vi "Package Builder.vi"() -> ()   [LabVIEW 2019, in "VIPM.lvclass"]
uses:
  VIPM.lvclass
  <vilib>/Utility/sysdir.llb/System Directory Type.ctl
  <vilib>/Utility/file.llb/Read Delimited Spreadsheet (string).vi
  <vilib>/Utility/file.llb/Write Delimited Spreadsheet (string).vi
  <vilib>/JKI/VIPM API/VIPM API_vipm_api.lvlib
panel:
  out "Package Builder":string
  in  "Clear Notes":bool
  in  "Release Notes":string
  in  "Append Notes":bool
  in  "ALL":bool
  in  "Patch +1":bool
  out "Selected File List":string
  in  "Publish":bool
  in  "Open List":bool
  in  "Build":bool
  in  "Preview":bool
  out "Status":string
  in  "File List":i32(listbox)
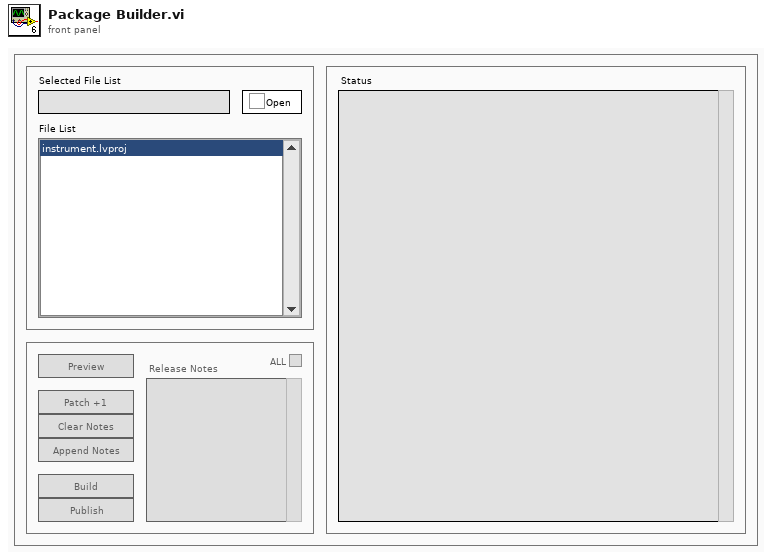
[diagram p1: front panel]
types:
  T1 = enum32{"Invalid", "Standard", "Closed", "Hidden", "Minimized", "Maximized"}
  T2 = enum32{"invalid app kind", "Development System", "Run Time System", "Student Edition", "Embedded LabVIEW", "Evaluation", "Custom"}
  T3 = enum8{"Enabled", "Disabled", "Disabled and Grayed Out"}
  T4 = cluster{"Core":cluster{"Current VI Reference":refnum<vi>, "Close Panel on Exit?":bool}, "lvproj paths":path[], "vipb paths":path[], "vip paths":path[], "selected path":path, "config path":path}
  T5 = typedef "System Directory Type.ctl" = i32
  T6 = cluster{"Current VI Reference":refnum<vi>, "Close Panel on Exit?":bool}
  T7 = typedef "VIPM API_vipm_api.lvlib/VI Package Build Spec Data Cluster_vipm_api.ctl" = cluster{"Package Version":T8, "Product Name":string, "Company Name":string, "Author Name (Person or Company)":string, "Product Homepage (URL)":string, "Legal Copyright":string, "License Agreement Name":string, "Product Description Summary":string, "Product Description":string, "Release Notes - Change Log":string}
  T8 = typedef "VIPM API_vipm_api.lvlib/Version Info Cluster_vipm_api.ctl" = cluster{"major":u32, "minor":u32, "patch":u32, "build":u32}
  T9 = typedef "VIPM API_vipm_api.lvlib/Repository Info Cluster_vipm_api.ctl" = cluster{"Repository Name":string, "Repository Folder Location":path}
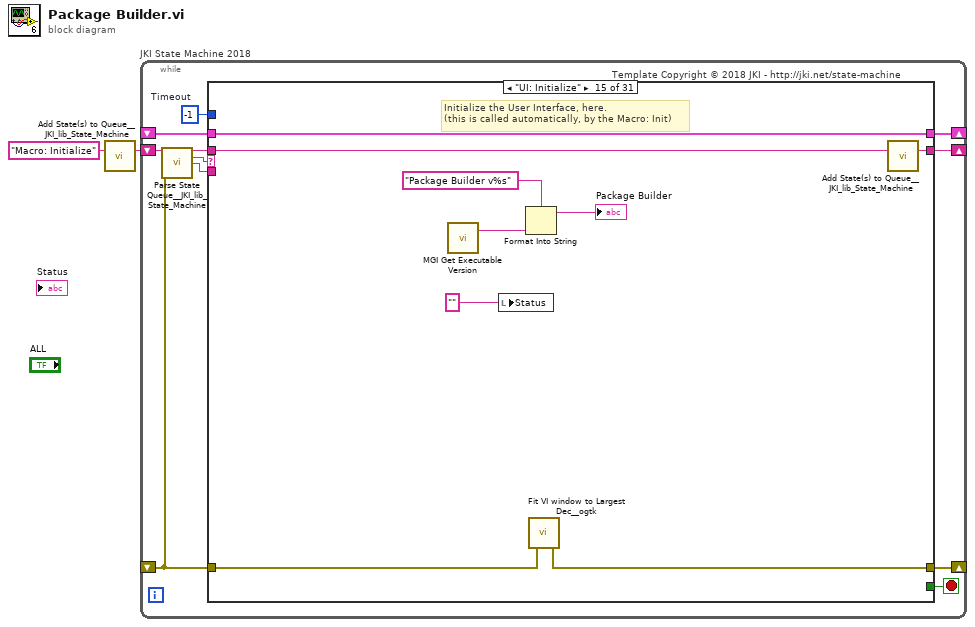
[diagram p0: block diagram]
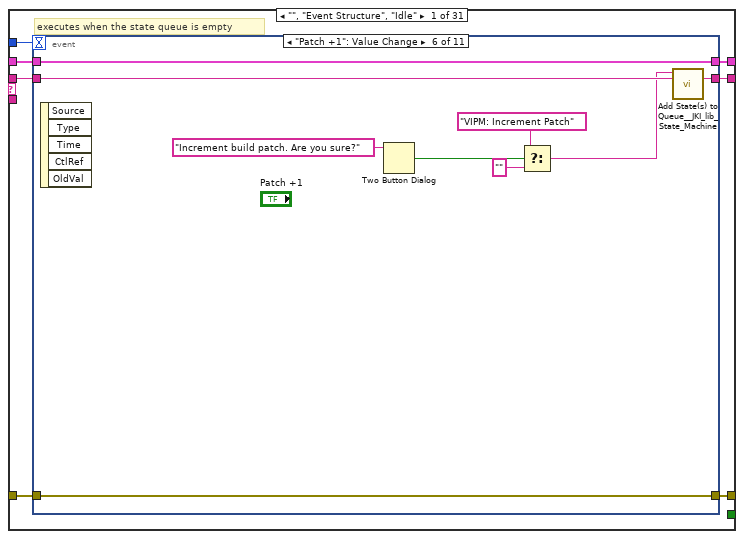
[diagram p2: hidden frame]
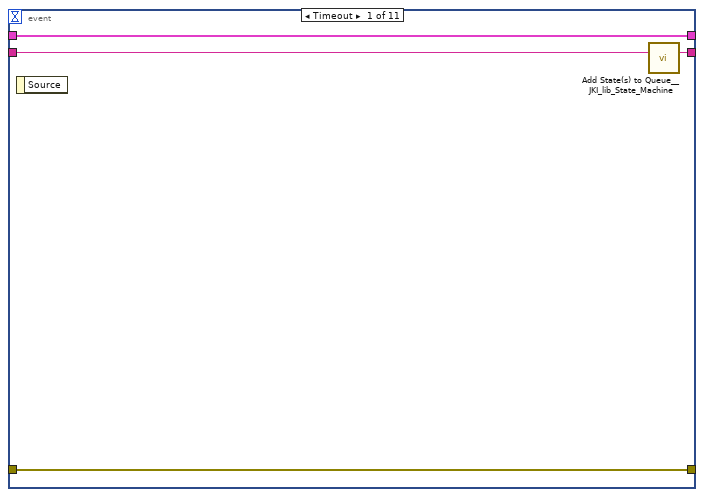
[diagram p3: hidden frame]
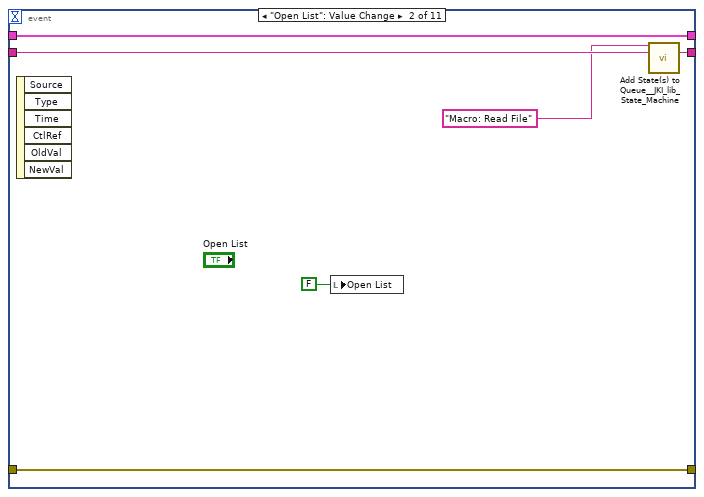
[diagram p4: hidden frame]
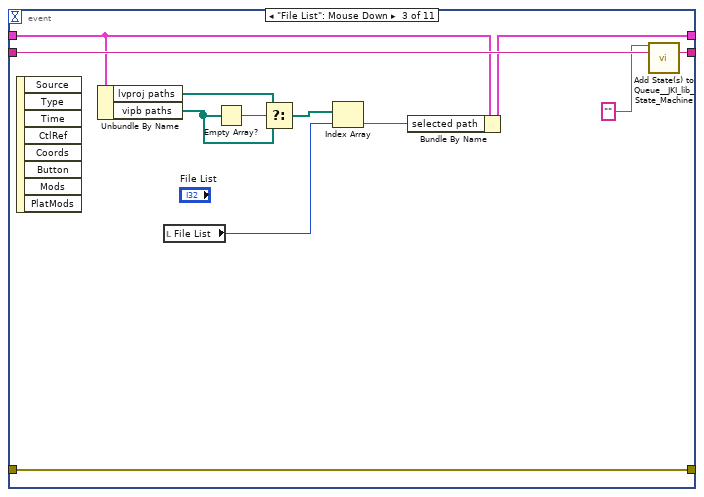
[diagram p5: hidden frame]
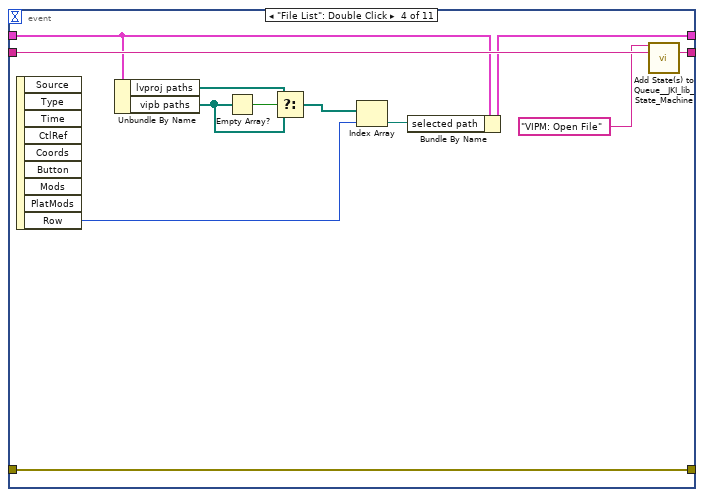
[diagram p6: hidden frame]
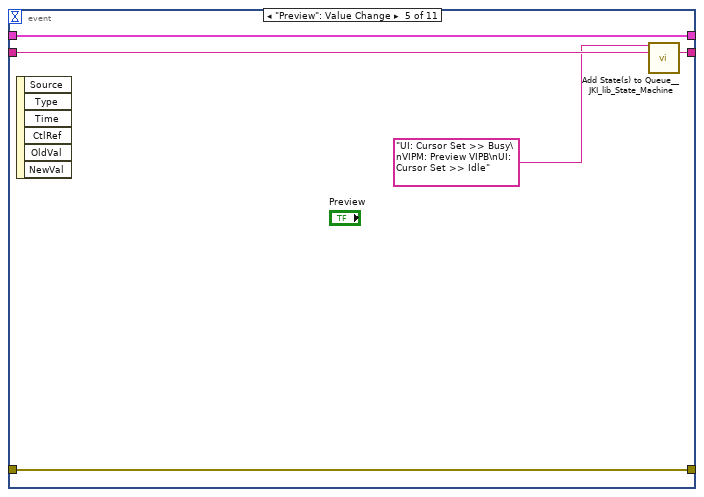
[diagram p7: hidden frame]
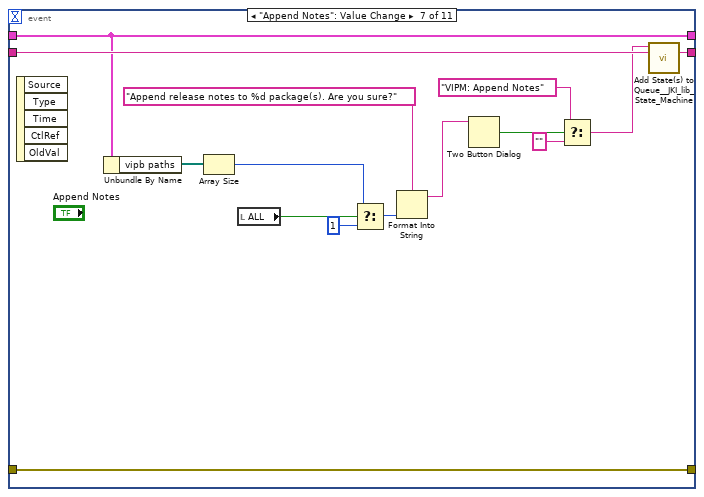
[diagram p8: hidden frame]
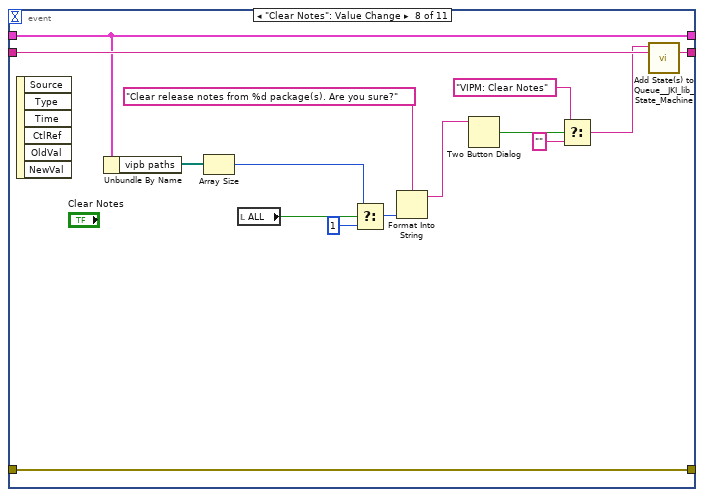
[diagram p9: hidden frame]
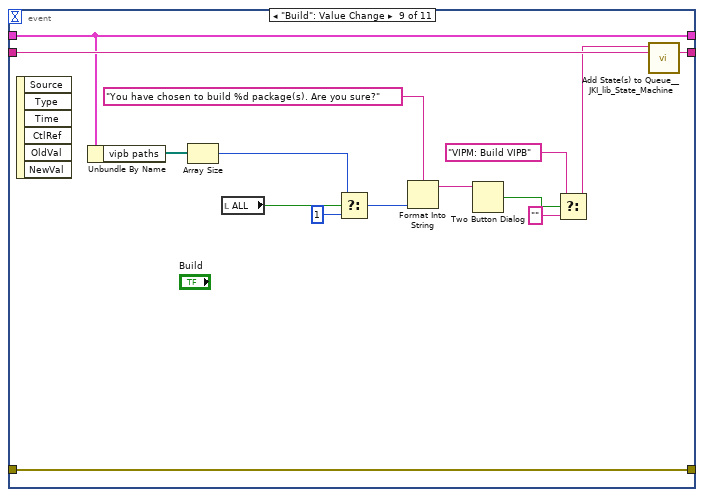
[diagram p10: hidden frame]
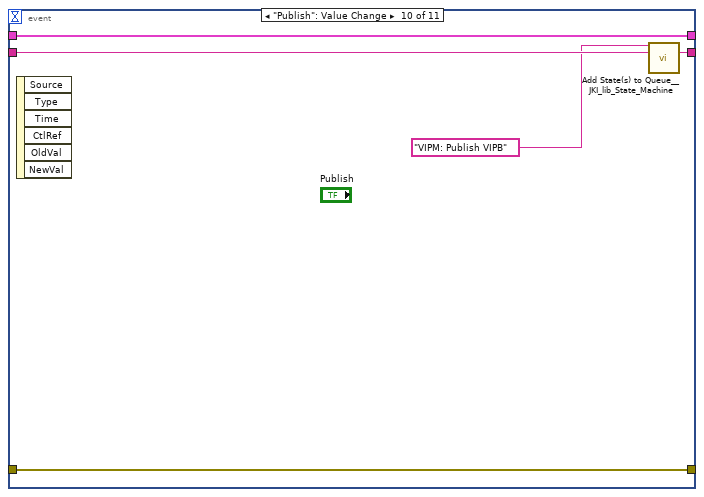
[diagram p11: hidden frame]
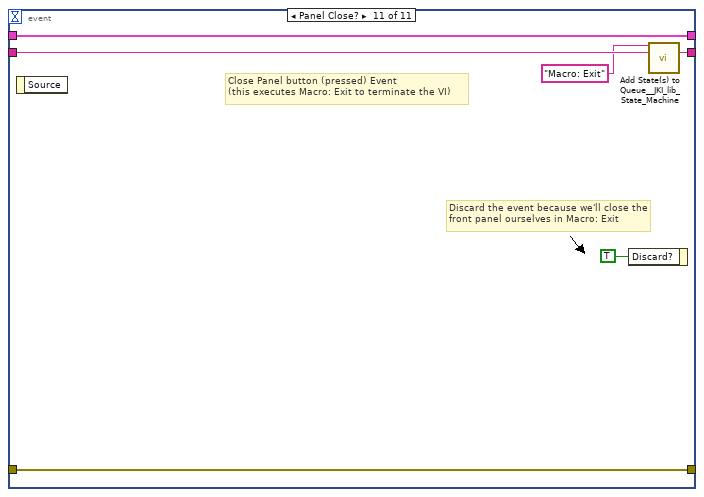
[diagram p12: hidden frame]
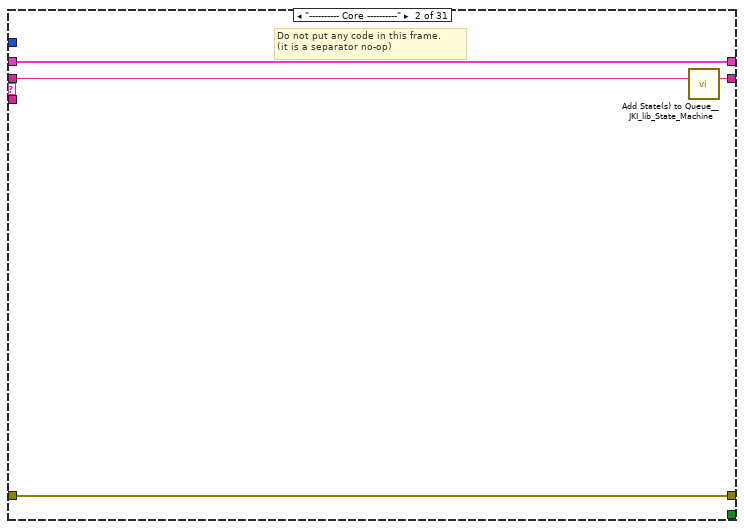
[diagram p13: hidden frame]
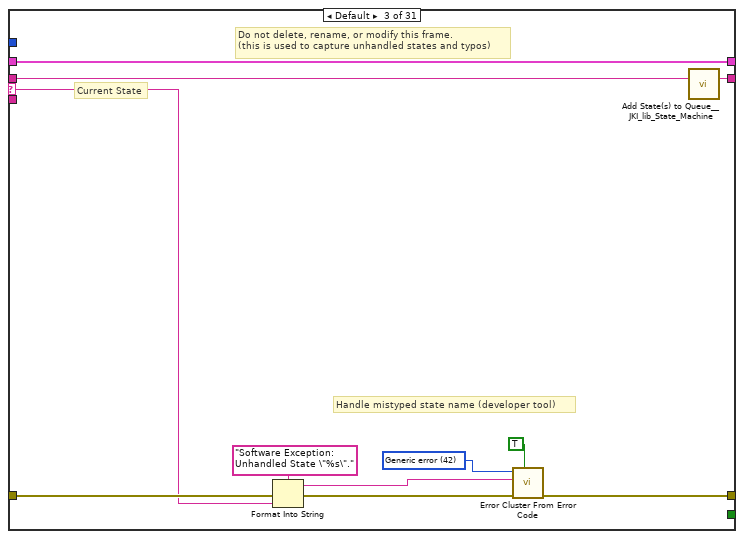
[diagram p14: hidden frame]
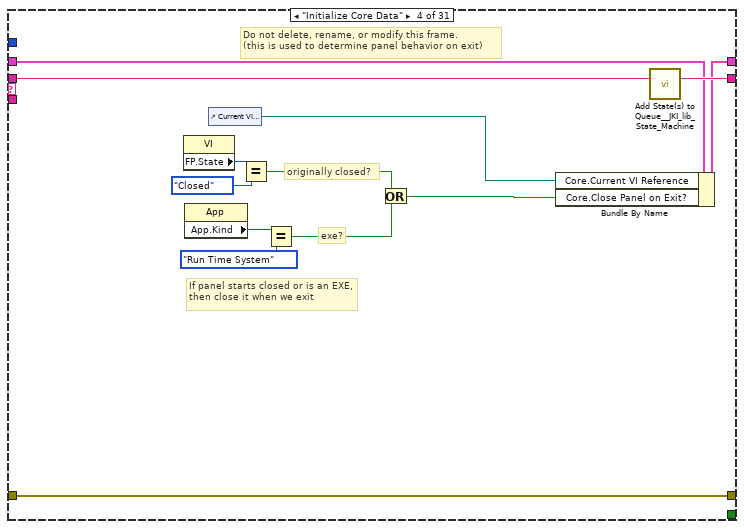
[diagram p15: hidden frame]
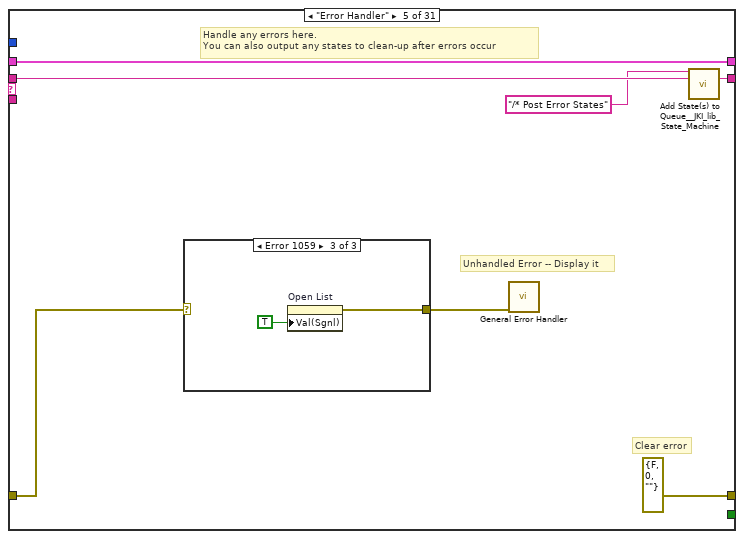
[diagram p16: hidden frame]
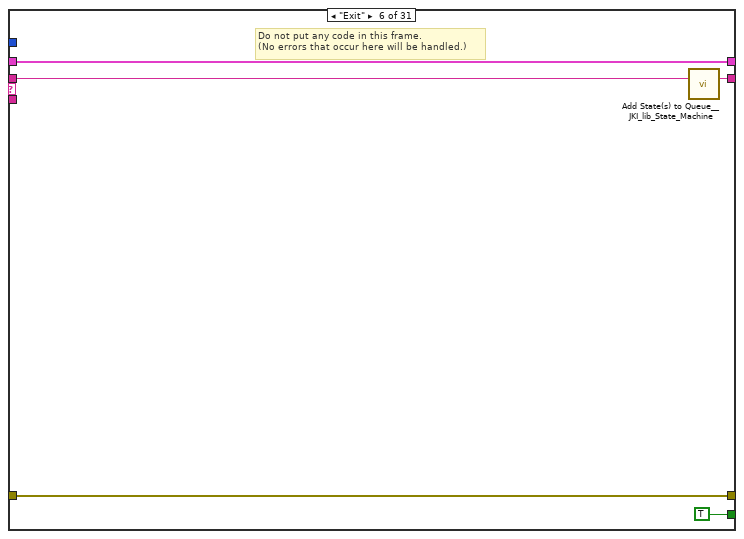
[diagram p19: hidden frame]
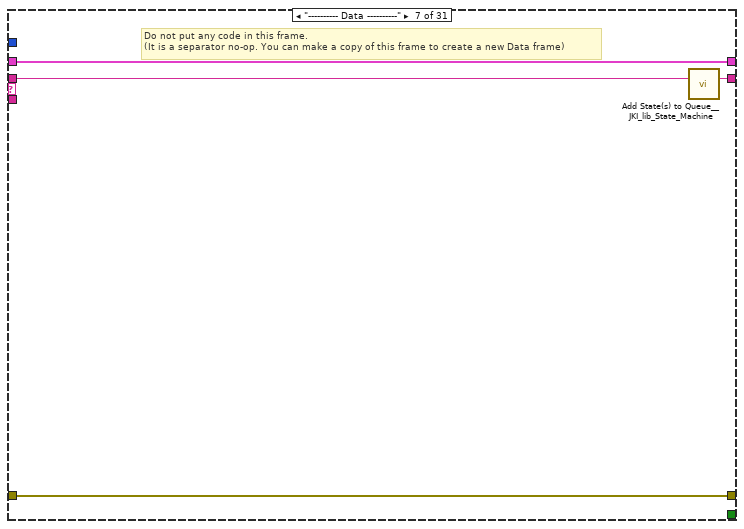
[diagram p20: hidden frame]
diagram:
  n1 = call <vilib>:"Add State(s) to Queue__JKI_lib_State_Machine.vi"("State(s) in (\"\")"="Macro: Initialize") -> ("States Out"=w2:string)  [unwired: 14 in]
  n2 = while "JKI State Machine 2018" {
    shift-right: [w6] -> _
    shift-left: _ -> [w5]
    shift-right: [w9] -> _
    shift-left: _ -> [w3]
    shift-right: [w8] -> _
    shift-left: w2 -> [w10]
    stop <- w7 stop-if-true
    w4 = -1  # Timeout
    # "Template Copyright © 2018 JKI - http://jki.net/state-machine"
    n3 = call <vilib>:"Parse State Queue__JKI_lib_State_Machine.vi"("State Queue"=w10, "Error In (no error)"=w3) -> ("Remaining States"=w12:string, "Current State"=w13:string, "Arguments"=w11:string)  [unwired: 11 in]
    n4 = case shown="\"UI: Initialize\"" w13 {
      selector: w13 -> [_ _ w129 _ _ _ _ _ _ _ _ _ _ _ _ _ _ _ _ _ _ _ _ _ _ _ _ _ _ _ _]
      tunnel: w12 -> [w20 w128 w133 w152 w159 w168 w172 w191 w197 w209 w222 w243 w262 w266 w275 w288 w305 w314 w325 w394 w399 w404 w414 w418 w431 w443 w462 w488 w512 w544 w561]
      tunnel: w11 -> [_ _ _ _ _ _ _ _ _ _ _ _ _ _ _ _ _ w309 w319 _ _ _ _ _ _ _ _ _ _ w532 _]
      tunnel: w5 -> [w18 w125 w131 w145 w156 w166 w169 _ w192 w201 w215 w240 w260 w263 w273 w285 w299 w312 w321 w391 w396 w401 w411 w415 w429 w441 w460 w486 w510 w535 w555]
      tunnel: [w17 w126 w135 w149 errorcluster {"status"=FALSE, "code"=0, "source"=""} ("error out") w165 w170 w183 w193 w207 w212 w229 w256 w264 w272 w286 w303 w310 w322 w392 w397 w402 w412 w416 w424 w440 w453 w479 w503 w538 w553] -> w9
      tunnel: w3 -> [w16 w126 w134 w149 w154 w165 w170 w182 w194 w207 w217 w238 w257 w264 w271 w286 w303 w311 w323 w392 w397 w402 w412 w416 w423 w439 w452 w478 w502 w537 w552]
      tunnel: [w19 w127 w132 w151 w158 w167 w171 w190 w196 w208 w221 w242 w261 w265 w274 w287 w304 w313 w324 w393 w398 w403 w413 w417 w430 w442 w461 w487 w511 w543 w560] -> w8
      tunnel: [_ _ _ _ _ TRUE _ _ _ _ _ _ _ _ _ _ _ _ _ _ _ _ _ _ _ _ _ _ _ _ _] -> w7
      tunnel: [w15 w125 w131 w150 w156 w166 w169 w189 w192 w202 w216 w241 w260 w263 w273 w285 w299 w312 w321 w391 w396 w401 w411 w415 w429 w441 w460 w486 w510 w536 w555] -> w6
      tunnel: w4 -> [w14 _ _ _ _ _ _ _ _ _ _ _ _ _ _ _ _ _ _ _ _ _ _ _ _ _ _ _ _ _ _]
      frame "", "Event Structure", "Idle" {
        # "executes when the state queue is empty"
        n5 = event shown="[5] \"Patch +1\": Value Change" {
          selector: _ -> [_ _ _ _ _ _ _ _ _ _ _]
          dyn-events: _ -> [_ _ _ _ _ _ _ _ _ _ _]
          timeout: w14 -> [_ _ _ _ _ _ _ _ _ _ _]
          tunnel: w20 -> [w24 w30 w42 w54 w59 w68 w83 w98 w113 w118 w124]
          tunnel: [w23 w29 w41 w53 w58 w67 w82 w97 w112 w117 w123] -> w19
          tunnel: w18 -> [w21 w25 w39 w44 w56 w65 w69 w84 w105 w115 w121]
          tunnel: [w22 w26 w40 w52 w57 w66 w81 w96 w111 w116 w122] -> w17
          tunnel: w16 -> [w22 w26 w40 w52 w57 w66 w81 w96 w111 w116 w122]
          tunnel: [w21 w25 w38 w51 w56 w65 w69 w84 w105 w115 w121] -> w15
          event Timeout {
            n6 = event-data() -> ()  [unwired: 1 in, 1 out]
            n7 = call <vilib>:"Add State(s) to Queue__JKI_lib_State_Machine.vi"("State(s) in (\"\")"=w24) -> ("States Out"=w23:string)  [unwired: 14 in]
          }
          event "Open List": Value Change {
            n8 = event-data() -> ()  [unwired: 1 in, 6 out]
            n9 = local write "Open List"(FALSE ("Choose File")) -> ()
            n10 = call <vilib>:"Add State(s) to Queue__JKI_lib_State_Machine.vi"("State(s) in Front (\"\")"="Macro: Read File" ("State(s) in Front (\"\")"), "State(s) in (\"\")"=w30) -> ("States Out"=w29:string)  [unwired: 13 in]
          }
          event "File List": Mouse Down {
            n11 = event-data() -> ()  [unwired: 1 in, 8 out]
            n12 = Unbundle By Name(w39) -> ("lvproj paths"=w33:path[], "vipb paths"=w31:path[])
            n13 = local read "File List"() -> (w35:i32)
            n14 = Empty Array?(array=w31) -> (empty?=w34:bool)
            n15 = Select(t=w33, s=w34, f=w31) -> (s? t:f=w32:path[])
            n16 = Index Array(array=w32, index=w35) -> (element=w37:path)
            n17 = Bundle By Name(cluster=w39, "selected path"=w37) -> (w38:T4)
            n18 = call <vilib>:"Add State(s) to Queue__JKI_lib_State_Machine.vi"("State(s) in Front (\"\")"="" ("State(s) in Front (\"\")"), "State(s) in (\"\")"=w42) -> ("States Out"=w41:string)  [unwired: 13 in]
          }
          event "File List": Double Click {
            n19 = event-data() -> ("Row"=w43:i32)  [unwired: 1 in, 8 out]
            n20 = Unbundle By Name(w44) -> ("lvproj paths"=w47:path[], "vipb paths"=w46:path[])
            n21 = Empty Array?(array=w46) -> (empty?=w48:bool)
            n22 = Select(t=w47, s=w48, f=w46) -> (s? t:f=w45:path[])
            n23 = Index Array(array=w45, index=w43) -> (element=w50:path)
            n24 = Bundle By Name(cluster=w44, "selected path"=w50) -> (w51:T4)
            n25 = call <vilib>:"Add State(s) to Queue__JKI_lib_State_Machine.vi"("State(s) in Front (\"\")"="VIPM: Open File" ("State(s) in Front (\"\")"), "State(s) in (\"\")"=w54) -> ("States Out"=w53:string)  [unwired: 13 in]
          }
          event "Preview": Value Change {
            n26 = event-data() -> ()  [unwired: 1 in, 6 out]
            n27 = call <vilib>:"Add State(s) to Queue__JKI_lib_State_Machine.vi"("State(s) in Front (\"\")"="UI: Cursor Set >> Busy\nVIPM: Preview VIPB\nUI: Cursor Set >> Idle" ("State(s) in Front (\"\")"), "State(s) in (\"\")"=w59) -> ("States Out"=w58:string)  [unwired: 13 in]
          }
          event "Patch +1": Value Change {
            n28 = event-data() -> ()  [unwired: 1 in, 5 out]
            n29 = Two Button Dialog(message="Increment build patch. Are you sure?") -> (T button?=w63:bool)  [unwired: 2 in]
            n30 = Select(t="VIPM: Increment Patch" ("State(s) in Front (\"\")"), s=w63, f="") -> (s? t:f=w60:string)
            n31 = call <vilib>:"Add State(s) to Queue__JKI_lib_State_Machine.vi"("State(s) in Front (\"\")"=w60, "State(s) in (\"\")"=w68) -> ("States Out"=w67:string)  [unwired: 13 in]
          }
          event "Append Notes": Value Change {
            n32 = event-data() -> ()  [unwired: 1 in, 5 out]
            n33 = Unbundle By Name(w69) -> ("vipb paths"=w76:path[])
            n34 = Array Size(array=w76) -> (size(s)=w74:i32)
            n35 = local read "ALL"() -> (w75:bool)
            n36 = Select(t=w74, s=w75, f=1) -> (s? t:f=w77:i32)
            n37 = Format Into String(format string="Append release notes to %d package(s). Are you sure?" ("message"), w77) -> (resulting string=w71:string)  [unwired: 2 in, 1 out]
            n38 = Two Button Dialog(message=w71) -> (T button?=w80:bool)  [unwired: 2 in]
            n39 = Select(t="VIPM: Append Notes" ("State(s) in Front (\"\")"), s=w80, f="") -> (s? t:f=w78:string)
            n40 = call <vilib>:"Add State(s) to Queue__JKI_lib_State_Machine.vi"("State(s) in Front (\"\")"=w78, "State(s) in (\"\")"=w83) -> ("States Out"=w82:string)  [unwired: 13 in]
          }
          event "Clear Notes": Value Change {
            n41 = event-data() -> ()  [unwired: 1 in, 6 out]
            n42 = Unbundle By Name(w84) -> ("vipb paths"=w91:path[])
            n43 = Array Size(array=w91) -> (size(s)=w89:i32)
            n44 = local read "ALL"() -> (w90:bool)
            n45 = Select(t=w89, s=w90, f=1) -> (s? t:f=w92:i32)
            n46 = Format Into String(format string="Clear release notes from %d package(s). Are you sure?" ("message"), w92) -> (resulting string=w86:string)  [unwired: 2 in, 1 out]
            n47 = Two Button Dialog(message=w86) -> (T button?=w95:bool)  [unwired: 2 in]
            n48 = Select(t="VIPM: Clear Notes" ("State(s) in Front (\"\")"), s=w95, f="") -> (s? t:f=w93:string)
            n49 = call <vilib>:"Add State(s) to Queue__JKI_lib_State_Machine.vi"("State(s) in Front (\"\")"=w93, "State(s) in (\"\")"=w98) -> ("States Out"=w97:string)  [unwired: 13 in]
          }
          event "Build": Value Change {
            n50 = event-data() -> ()  [unwired: 1 in, 6 out]
            n51 = Unbundle By Name(w105) -> ("vipb paths"=w104:path[])
            n52 = Array Size(array=w104) -> (size(s)=w102:i32)
            n53 = local read "ALL"() -> (w103:bool)
            n54 = Select(t=w102, s=w103, f=1) -> (s? t:f=w100:i32)
            n55 = Format Into String(format string="You have chosen to build %d package(s). Are you sure?" ("message"), w100) -> (resulting string=w99:string)  [unwired: 2 in, 1 out]
            n56 = Two Button Dialog(message=w99) -> (T button?=w109:bool)  [unwired: 2 in]
            n57 = Select(t="VIPM: Build VIPB" ("State(s) in Front (\"\")"), s=w109, f="") -> (s? t:f=w106:string)
            n58 = call <vilib>:"Add State(s) to Queue__JKI_lib_State_Machine.vi"("State(s) in Front (\"\")"=w106, "State(s) in (\"\")"=w113) -> ("States Out"=w112:string)  [unwired: 13 in]
          }
          event "Publish": Value Change {
            n59 = event-data() -> ()  [unwired: 1 in, 6 out]
            n60 = call <vilib>:"Add State(s) to Queue__JKI_lib_State_Machine.vi"("State(s) in Front (\"\")"="VIPM: Publish VIPB" ("State(s) in Front (\"\")"), "State(s) in (\"\")"=w118) -> ("States Out"=w117:string)  [unwired: 13 in]
          }
          event Panel Close? {
            # "Discard the event because we'll close the front panel ourselves in Macro: Exit"
            # "Close Panel button (pressed) Event\n(this executes Macro: Exit to terminate the VI)"
            n61 = event-data() -> ()  [unwired: 1 in, 1 out]
            n62 = event-data("Discard?"=TRUE) -> ()  [unwired: 1 in, 1 out]
            n63 = call <vilib>:"Add State(s) to Queue__JKI_lib_State_Machine.vi"("State(s) in Front (\"\")"="Macro: Exit", "State(s) in (\"\")"=w124) -> ("States Out"=w123:string)  [unwired: 13 in]
          }
        }
      }
      frame "---------- Core ----------" {
        # "Do not put any code in this frame.\n(it is a separator no-op)"
        n64 = call <vilib>:"Add State(s) to Queue__JKI_lib_State_Machine.vi"("State(s) in (\"\")"=w128) -> ("States Out"=w127:string)  [unwired: 14 in]
      }
      frame Default {
        w138 = 42 items=["No error", "Argument error", "Memory is full", "Out of zone", "End of file", "File already open", "Generic file I/O error", "File not found", "File permission error", "Disk is full", "Duplicate path", "Too many files open", "System feature not enabled", "Resource file not found", "Cannot add resource", "Resource not found", "Image not found", "Image memory error", "Pen does not exist", "Config type invalid", "Config token not found", "Config parse error", "Config memory error", "Bad external code format", "Bad external code offset", "External code not present", "Null window", "Destroy window error", "Null menu", "Print aborted", "Bad print record", "Print driver error", "Windows error during printing", "Memory error during printing", "Print dialog error", "Generic print error", "Invalid device refnum", "Device not found", "Device parameter error", "Device unit error", "Cannot open device", "Device call aborted", "Generic error", "Cancelled by user", "Object ID too low", "Object ID too high", "Object not in heap", "Unknown heap", "Unknown object (invalid DefProc)", "Unknown object (DefProc not in table)", "Message out of range", "Invalid (null) method", "Unknown message", "Manager call not supported", "Bad address", "Network operation in progress", "Network operation timed out", "Connection is busy", "Network attribute not supported", "Network error", "Address in use", "System out of memory", "Connection aborted", "Connection refused", "Not connected", "Already connected", "Connection closed", "Initialization error (interapplication manager)", "Bad occurrence", "Wait on unbound occurrence handler", "Occurrence queue overflow", "Datalog type conflict", "Unused", "Unrecognized type (interapplication manager)", "Memory corrupt", "Failed to make temporary DLL", "Old CIN version", "Drag socket not found", "Failed to load drop-object", "Failed to register OLE object", "Failed to release OLE object", "Format specifier type mismatch", "Unknown format specifier", "Too few format specifiers", "Too many format specifiers", "Scan failed", "Newer CIN version", "Error converting to variant", "Runtime menu error", "Password tampered", "Variant attribute not found", "Incompatible variant data type", "Event data is not available", "Event Store is not present", "Occurrence is not found", "Event Queue is not created", "Event info is not available", "Refnum passed is NULL", "Error retrieving Class GUID", "Error retrieving CoClass GUID", "Error retrieving TypeLib GUID.", "Bad built application magic bytes.", "Specific driver is different from the specific driver associated with the Logical Name.", "There is no session opened to the class driver.", "Max Error", "MAX - Error with config objects", "MAX - Error loading configuration", "MAX - Group not supported"]
        # "Current State"
        # "Do not delete, rename, or modify this frame.\n(this is used to capture unhandled states and typos)"
        # "Handle mistyped state name (developer tool)"
        n65 = Format Into String(format string="Software Exception: Unhandled State \"%s\"." ("message"), error in=w134, w129) -> (resulting string=w137:string, error out=w136:errorcluster)  [unwired: 1 in]
        n66 = call <vilib>:"Error Cluster From Error Code.vi"("show call chain? (False)"=TRUE, "error in (no error)"=w136, "error message (\"\")"=w137, "error code (0)"=w138) -> ("error out"=w135:errorcluster)  [unwired: 5 in]
        n67 = call <vilib>:"Add State(s) to Queue__JKI_lib_State_Machine.vi"("State(s) in (\"\")"=w133) -> ("States Out"=w132:string)  [unwired: 14 in]
      }
      frame "Initialize Core Data" {
        # "Do not delete, rename, or modify this frame.\n(this is used to determine panel behavior on exit)"
        # "originally closed?"
        # "exe?"
        # "If panel starts closed or is an EXE, then close it when we exit"
        n68 = property class="VI"() -> ("FP.State"=w142:T1)  [unwired: 2 in, 2 out]
        n69 = property class="App"() -> ("App.Kind"=w148:T2)  [unwired: 2 in, 2 out]
        n70 = control-ref of="Current VI Reference"() -> (w143:refnum<vi>)
        n71 = Equal?(x=w142, y=T1."Closed" ("Front Panel Window:State")) -> (x = y?=w140:bool)
        n72 = Equal?(x=w148, y=T2."Run Time System" ("Application:Kind")) -> (x = y?=w146:bool)
        n73 = Or(x=w140, y=w146) -> (x .or. y?=w144:bool)
        n74 = Bundle By Name(cluster=w145, "Core.Current VI Reference"=w143, "Core.Close Panel on Exit?"=w144) -> (w150:T4)
        n75 = call <vilib>:"Add State(s) to Queue__JKI_lib_State_Machine.vi"("State(s) in (\"\")"=w152) -> ("States Out"=w151:string)  [unwired: 14 in]
      }
      frame "Error Handler" {
        # "Unhandled Error -- Display it"
        # "Handle any errors here.\nYou can also output any states to clean-up after errors occur"
        # "Clear error"
        n76 = case shown="Error 1059" w154 {
          selector: w154 -> [w160 w161 _]
          tunnel: [w160 w161 w162] -> w153
          frame No Error {
          }
          frame Default {
          }
          frame Error {
            n77 = property on="Open List" class="Bool (strict)"("Val(Sgnl)"=TRUE) -> (error out=w162:errorcluster)  [unwired: 2 in, 1 out]
          }
        }
        n78 = call <vilib>:"General Error Handler.vi"("error in (no error)"=w153) -> ()  [unwired: 10 in, 5 out]
        n79 = call <vilib>:"Add State(s) to Queue__JKI_lib_State_Machine.vi"("State(s) in Front (\"\")"="/* Post Error States", "State(s) in (\"\")"=w159) -> ("States Out"=w158:string)  [unwired: 13 in]
      }
      frame "Exit" {
        # "Do not put any code in this frame.\n(No errors that occur here will be handled.)"
        n80 = call <vilib>:"Add State(s) to Queue__JKI_lib_State_Machine.vi"("State(s) in (\"\")"=w168) -> ("States Out"=w167:string)  [unwired: 14 in]
      }
      frame "---------- Data ----------" {
        # "Do not put any code in this frame.\n(It is a separator no-op. You can make a copy of this frame to create a new Data frame)"
        n81 = call <vilib>:"Add State(s) to Queue__JKI_lib_State_Machine.vi"("State(s) in (\"\")"=w172) -> ("States Out"=w171:string)  [unwired: 14 in]
      }
      frame "Data: Initialize" {
        w178 = T5 3 items=["User Home"=0, "User Desktop"=1, "User Documents"=2, "User Application Data"=3, "User Preferences"=4, "User Temporary"=5, "Public Documents"=6, "Public Application Data"=7, "Public Preferences"=8, "Public Cache"=13, "System Core Libraries"=9, "System Installed Libraries"=10, "Application Files"=11, "Boot Volume Root"=12] ("system directory type")
        w179 = path[] []  # lvproj paths
        w180 = path[] []  # vip paths
        w181 = path[] []  # vipb paths
        w185 = path ""  # config path
        w187 = path ""  # selected path
        w188 = T6 {"Current VI Reference"=refnum, "Close Panel on Exit?"=FALSE}  # Core
        # "Initialize the shift-register data, here.\n(data names are defined by what you wire into the bundle function)"
        n82 = call <vilib>:"Get System Directory.vi"("system directory type"=w178) -> ("system directory"=w175:path)  [unwired: 10 in]
        n83 = Build Path(base path=w175, name or relative path="LevyLab") -> (appended path=w174:path)
        n84 = Build Path(base path=w174, name or relative path="build-support") -> (appended path=w176:path)
        n85 = call <userlib>:"Create Dir if Non-Existant__ogtk.vi"("error in (no error)"=w182, "Directory Path"=w176) -> ("error out"=w183:errorcluster, "dup Directory Path"=w184:path)  [unwired: 7 in, 1 out]
        n86 = Variant To Data(type=w185, Variant=w184) -> (data=w186:path)  [unwired: 1 in, 1 out]
        n87 = Bundle("Core"=w188, "lvproj paths"=w179, "vipb paths"=w181, "vip paths"=w180, "selected path"=w187, "config path"=w186) -> (w189:T4)  [unwired: 1 in]
        n88 = call <vilib>:"Add State(s) to Queue__JKI_lib_State_Machine.vi"("State(s) in (\"\")"=w191) -> ("States Out"=w190:string)  [unwired: 14 in]
      }
      frame "Data: Cleanup" {
        # "Cleanup any data and references, here.\n(this is called automatically, by the Macro: Exit)"
        n89 = Unbundle By Name(w192) -> ("Core.Current VI Reference"=w195:refnum<vi>)
        n90 = Close Reference(reference=w195, error in (no error)=w194) -> (error out=w193:errorcluster)
        n91 = call <vilib>:"Add State(s) to Queue__JKI_lib_State_Machine.vi"("State(s) in (\"\")"=w197) -> ("States Out"=w196:string)  [unwired: 14 in]
      }
      frame "Data: Update Listbox" {
        w198 = 0 ("Value (Signaling)")
        # "Do not put any code in this frame.\n(It is a separator no-op. You can make a copy of this frame to create a new Data frame)"
        n92 = Unbundle By Name(w201) -> ("lvproj paths"=w204:path[], "vipb paths"=w203:path[])
        n93 = Empty Array?(array=w203) -> (empty?=w205:bool)
        n94 = Select(t=w204, s=w205, f=w203) -> (s? t:f=w200:path[])
        n95 = for {
          tunnel: w200 -> [w211] mode=indexing
          tunnel: [w210] -> w206 mode=indexing
          n96 = Strip Path(path=w211) -> (name=w210:string)  [unwired: 1 out]
        }
        n97 = property on="File List" class="LstBox (strict)"("Item Names"=w206, "Val(Sgnl)"=w198) -> ()  [unwired: 2 in, 2 out]
        n98 = Index Array(array=w200, index=w198) -> (element=w199:path)
        n99 = Bundle By Name(cluster=w201, "selected path"=w199) -> (w202:T4)
        n100 = call <vilib>:"Add State(s) to Queue__JKI_lib_State_Machine.vi"("State(s) in (\"\")"=w209) -> ("States Out"=w208:string)  [unwired: 14 in]
      }
      frame "Data: Choose Config File" {
        # "Do not put any code in this frame.\n(It is a separator no-op. You can make a copy of this frame to create a new Data frame)"
        n101 = Unbundle By Name(w215) -> ("config path"=w220:path)
        n102 = call "File Dialog"("start path"=w220, "error in"=w217) -> ("selected path"=w219:path, "cancelled"=w214:bool, "error out"=w213:errorcluster)  [unwired: 10 in, 1 out]
        n103 = case shown="False" w214 {
          tunnel: w219 -> [w223 _]
          tunnel: [w227 _] -> w218
          tunnel: [w226 w228] -> w216
          tunnel: w215 -> [w225 w228]
          tunnel: w213 -> [w224 _]
          tunnel: [w224 _] -> w212
          frame False {
            n104 = Bundle By Name(cluster=w225, "config path"=w223) -> (w226:T4)
            n105 = Strip Path(path=w223) -> (name=w227:string)  [unwired: 1 out]
          }
          frame True {
          }
        }
        "Selected File List" <- w218
        n106 = call <vilib>:"Add State(s) to Queue__JKI_lib_State_Machine.vi"("State(s) in (\"\")"=w222) -> ("States Out"=w221:string)  [unwired: 14 in]
      }
      frame "Data: Read Config File" {
        (unwired) 0 ("disabled index (col)")
        # "Do not put any code in this frame.\n(It is a separator no-op. You can make a copy of this frame to create a new Data frame)"
        n107 = Unbundle By Name(w240) -> ("config path"=w239:path)
        n108 = call-poly <vilib>:"Read Delimited Spreadsheet.vi"("file path (dialog if empty)"=w239, "error in (no error)"=w238, "transpose? (F)"=TRUE, "delimiter (\\t)"="\\n" ("delimiter (\\t)")) -> ("all rows"=w236:string[][], "error out"=w230:errorcluster)  [unwired: 6 in, 4 out]
        n109 = Index Array(array=w236) -> (element=w235:string[])  [unwired: 2 in]
        n110 = String To Path(string=w235) -> (path=w233:path[])
        n111 = for {
          tunnel: w233 -> [w252] mode=indexing
          tunnel: [w247] -> w232 mode=indexing if=w250
          tunnel: [w247] -> w231 mode=indexing if=w246
          tunnel: w230 -> [w245]
          tunnel: [w244] -> w229
          n112 = call <vilib>:"Get File Extension.vi"("error in (no error)"=w245, "file"=w252) -> ("error out"=w244:errorcluster, "lowercase file extension"=w248:string, "dup file"=w247:path)  [unwired: 5 in, 2 out]
          n113 = Equal?(x=w248, y="vipb") -> (x = y?=w250:bool)
          n114 = Equal?(x=w248, y="lvproj") -> (x = y?=w246:bool)
        }
        n115 = Bundle By Name(cluster=w240, "vipb paths"=w232, "lvproj paths"=w231) -> (w241:T4)
        n116 = call <vilib>:"Add State(s) to Queue__JKI_lib_State_Machine.vi"("State(s) in (\"\")"=w243) -> ("States Out"=w242:string)  [unwired: 14 in]
      }
      frame "Data: Write Config File" {
        # "Do not put any code in this frame.\n(It is a separator no-op. You can make a copy of this frame to create a new Data frame)"
        n117 = Unbundle By Name(w260) -> ("config path"=w255:path, "vipb paths"=w259:path[])
        n118 = Path To String(path=w259) -> (string=w258:string[])
        n119 = call-poly <vilib>:"Write Delimited Spreadsheet.vi"("file path (dialog if empty)"=w255, "1D data"=w258, "error in (no error)"=w257, "transpose? (no:F)"=TRUE, "delimiter (\\t)"="\\n" ("delimiter (\\t)")) -> ("error out"=w256:errorcluster)  [unwired: 9 in, 1 out]
        n120 = call <vilib>:"Add State(s) to Queue__JKI_lib_State_Machine.vi"("State(s) in (\"\")"=w262) -> ("States Out"=w261:string)  [unwired: 14 in]
      }
      frame "---------- UI ----------" {
        # "Do not put any code in this frame.\n(It is a separator no-op. You can make a copy of this frame to create a new UI frame)"
        n121 = call <vilib>:"Add State(s) to Queue__JKI_lib_State_Machine.vi"("State(s) in (\"\")"=w266) -> ("States Out"=w265:string)  [unwired: 14 in]
      }
      frame "UI: Initialize" {
        # "Initialize the User Interface, here.\n(this is called automatically, by the Macro: Init)"
        n122 = call <userlib>:"MGI Get Executable Version.vi"() -> ("Version"=w268:string)  [unwired: 7 in]
        n123 = local write "Status"("" ("Status")) -> ()
        n124 = Format Into String(format string="Package Builder v%s", w268) -> (resulting string=→"Package Builder":string)  [unwired: 2 in, 1 out]
        n125 = call <userlib>:"Fit VI window to Largest Dec__ogtk.vi"("error in (no error)"=w271) -> ("error out"=w272:errorcluster)  [unwired: 5 in, 1 out]
        n126 = call <vilib>:"Add State(s) to Queue__JKI_lib_State_Machine.vi"("State(s) in (\"\")"=w275) -> ("States Out"=w274:string)  [unwired: 14 in]
      }
      frame "UI: Disable Buttons" {
        # "Do not put any code in this frame.\n(It is a separator no-op. You can make a copy of this frame to create a new UI frame)"
        n127 = control-ref of="Preview"() -> (w284:refnum<vi>)
        n128 = control-ref of="Build"() -> (w283:refnum<vi>)
        n129 = control-ref of="Publish"() -> (w281:refnum<vi>)
        n130 = control-ref of="Clear Notes"() -> (w280:refnum<vi>)
        n131 = control-ref of="Append Notes"() -> (w279:refnum<vi>)
        n132 = control-ref of="Patch +1"() -> (w278:refnum<vi>)
        n133 = control-ref of="Release Notes"() -> (w277:refnum<vi>)
        n134 = control-ref of="ALL"() -> (w276:refnum<vi>)
        n135 = Build Array(w284, w283, w281, w280, w279, w278, w277, w276) -> (w282:refnum<vi>[])
        n136 = for {
          tunnel: w282 -> [w289] mode=indexing
          n137 = property class="Ctl"(reference=w289, "DisabledEnum"=T3."Disabled and Grayed Out" ("Disabled")) -> ()  [unwired: 1 in, 2 out]
        }
        n138 = call <vilib>:"Add State(s) to Queue__JKI_lib_State_Machine.vi"("State(s) in (\"\")"=w288) -> ("States Out"=w287:string)  [unwired: 14 in]
      }
      frame "UI: Enable Buttons" {
        # "Do not put any code in this frame.\n(It is a separator no-op. You can make a copy of this frame to create a new UI frame)"
        n139 = Unbundle By Name(w299) -> ("vipb paths"=w300:path[])
        n140 = control-ref of="Preview"() -> (w302:refnum<vi>)
        n141 = control-ref of="Build"() -> (w301:refnum<vi>)
        n142 = control-ref of="Publish"() -> (w298:refnum<vi>)
        n143 = control-ref of="Clear Notes"() -> (w297:refnum<vi>)
        n144 = control-ref of="Append Notes"() -> (w296:refnum<vi>)
        n145 = control-ref of="Patch +1"() -> (w293:refnum<vi>)
        n146 = control-ref of="Release Notes"() -> (w292:refnum<vi>)
        n147 = control-ref of="ALL"() -> (w291:refnum<vi>)
        n148 = Empty Array?(array=w300) -> (empty?=w294:bool)
        n149 = Build Array(w302, w301, w298, w297, w296, w293, w292, w291) -> (w295:refnum<vi>[])
        n150 = case shown="False" w294 {
          tunnel: w295 -> [w306 _]
          frame False {
            n151 = for {
              tunnel: w306 -> [w307] mode=indexing
              n152 = property class="Ctl"(reference=w307, "DisabledEnum"=T3."Enabled" ("Disabled")) -> ()  [unwired: 1 in, 2 out]
            }
          }
          frame True {
          }
        }
        n153 = call <vilib>:"Add State(s) to Queue__JKI_lib_State_Machine.vi"("State(s) in (\"\")"=w305) -> ("States Out"=w304:string)  [unwired: 14 in]
      }
      frame "UI: Cursor Set" {
        # "Argument"
        # "Set and Unset Cursor Busy.\n(Usage: \"UI: Cursor Set >> Busy|Idle\")"
        n154 = case shown="\"Idle\", Default" w309 {
          tunnel: w311 -> [w316 w318]
          tunnel: [w315 w317] -> w310
          frame "Idle", Default {
            n155 = call <vilib>:"Unset Busy.vi"("error in (no error)"=w316) -> ("error out"=w315:errorcluster)  [unwired: 10 in]
          }
          frame "Busy" {
            n156 = call <vilib>:"Set Busy.vi"("error in (no error)"=w318) -> ("error out"=w317:errorcluster)  [unwired: 9 in, 1 out]
          }
        }
        n157 = call <vilib>:"Add State(s) to Queue__JKI_lib_State_Machine.vi"("State(s) in (\"\")"=w314) -> ("States Out"=w313:string)  [unwired: 14 in]
      }
      frame "UI: Front Panel State" {
        # "Argument"
        # "Set Front Panel Open or Closed\n(Usage: \"UI: Front Panel State >> Open|Close\")"
        n158 = Unbundle By Name(w321) -> ("Core.Current VI Reference"=w320:refnum<vi>)
        n159 = case shown="\"Minimize\", \"Minimized\"" w319 {
          tunnel: w323 -> [w331 w346 w357 w370 w383]
          tunnel: [w333 w347 w359 w372 w385] -> w322
          tunnel: w320 -> [w332 w344 w358 w371 w384]
          frame "Open", "Standard", Default {
            w326 = T1."Standard" ("State")
            n160 = property class="VI"(reference=w332, error in=w331) -> (reference out=w329:refnum<vi>, error out=w330:errorcluster, "FP.State"=w328:T1)
            n161 = Not Equal?(x=w328, y=w326) -> (x != y?=w327:bool)
            n162 = case shown="True" w327 {
              tunnel: [w337 w339] -> w333
              tunnel: w330 -> [w336 w339]
              tunnel: w329 -> [w335 _]
              tunnel: w326 -> [w334 _]
              frame True {
                n163 = invoke class="VI" method="FP.Open"(reference=w335, error in=w336, "Activate"=TRUE, "State"=w334) -> (error out=w337:errorcluster)  [unwired: 1 in, 4 out]
              }
              frame False {
              }
            }
          }
          frame "Close", "Closed" {
            n164 = property class="VI"(reference=w344, error in=w346) -> (reference out=w343:refnum<vi>, error out=w345:errorcluster, "FP.State"=w341:T1)
            n165 = Not Equal?(x=w341, y=T1."Closed" ("Front Panel Window:State")) -> (x != y?=w340:bool)
            n166 = case shown="True" w340 {
              tunnel: [w348 w351] -> w347
              tunnel: w345 -> [w348 w350]
              tunnel: w343 -> [_ w349]
              frame False {
              }
              frame True {
                n167 = invoke class="VI" method="FP.Close"(reference=w349, error in=w350) -> (error out=w351:errorcluster)  [unwired: 1 in, 2 out]
              }
            }
          }
          frame "Hidden", "Hide" {
            w352 = T1."Hidden" ("State")
            n168 = property class="VI"(reference=w358, error in=w357) -> (reference out=w355:refnum<vi>, error out=w356:errorcluster, "FP.State"=w354:T1)
            n169 = Not Equal?(x=w354, y=w352) -> (x != y?=w353:bool)
            n170 = case shown="True" w353 {
              tunnel: [w363 w364] -> w359
              tunnel: w356 -> [w362 w364]
              tunnel: w355 -> [w361 _]
              tunnel: w352 -> [w360 _]
              frame True {
                n171 = invoke class="VI" method="FP.Open"(reference=w361, error in=w362, "State"=w360) -> (error out=w363:errorcluster)  [unwired: 2 in, 4 out]
              }
              frame False {
              }
            }
          }
          frame "Minimize", "Minimized" {
            w365 = T1."Minimized" ("State")
            n172 = property class="VI"(reference=w371, error in=w370) -> (reference out=w368:refnum<vi>, error out=w369:errorcluster, "FP.State"=w367:T1)
            n173 = Not Equal?(x=w367, y=w365) -> (x != y?=w366:bool)
            n174 = case shown="True" w366 {
              tunnel: [w376 w377] -> w372
              tunnel: w369 -> [w375 w377]
              tunnel: w368 -> [w374 _]
              tunnel: w365 -> [w373 _]
              frame True {
                n175 = invoke class="VI" method="FP.Open"(reference=w374, error in=w375, "State"=w373) -> (error out=w376:errorcluster)  [unwired: 2 in, 4 out]
              }
              frame False {
              }
            }
          }
          frame "Maximize", "Maximized" {
            w378 = T1."Maximized" ("State")
            n176 = property class="VI"(reference=w384, error in=w383) -> (reference out=w381:refnum<vi>, error out=w382:errorcluster, "FP.State"=w380:T1)
            n177 = Not Equal?(x=w380, y=w378) -> (x != y?=w379:bool)
            n178 = case shown="True" w379 {
              tunnel: [w389 w390] -> w385
              tunnel: w382 -> [w388 w390]
              tunnel: w381 -> [w387 _]
              tunnel: w378 -> [w386 _]
              frame True {
                n179 = invoke class="VI" method="FP.Open"(reference=w387, error in=w388, "State"=w386) -> (error out=w389:errorcluster)  [unwired: 2 in, 4 out]
              }
              frame False {
              }
            }
          }
        }
        n180 = call <vilib>:"Add State(s) to Queue__JKI_lib_State_Machine.vi"("State(s) in (\"\")"=w325) -> ("States Out"=w324:string)  [unwired: 14 in]
      }
      frame "---------- Macro ----------" {
        # "Do not put any code in this frame.\n(It is a separator no-op. You can make a copy of this frame to create a new Macro frame)"
        n181 = call <vilib>:"Add State(s) to Queue__JKI_lib_State_Machine.vi"("State(s) in (\"\")"=w394) -> ("States Out"=w393:string)  [unwired: 14 in]
      }
      frame "Macro: Initialize" {
        w395 = "Data: Initialize\nInitialize Core Data\nUI: Initialize\nUI: Front Panel State >> Open\n\nMacro: Read File"  # Data: Initialize Initialize Core Data UI: Initialize UI: Front Panel State >> Open  Macro: Read File
        # "Initialization Macro\n(This is called once, when the VI starts)"
        n182 = call <vilib>:"Add State(s) to Queue__JKI_lib_State_Machine.vi"("State(s) in Front (\"\")"=w395, "State(s) in (\"\")"=w399) -> ("States Out"=w398:string)  [unwired: 13 in]
      }
      frame "Macro: Read File" {
        w400 = "UI: Cursor Set >> Busy\nUI: Disable Buttons\nData: Choose Config File\nData: Read Config File\nData: Update Listbox\nUI: Enable Buttons\nUI: Cursor Set >> Idle"  # UI: Cursor Set >> Busy UI: Disable Buttons Data: Choose Config File Data: Read Config File Data: Update Listbox UI: Enable Buttons UI: Cursor Set >> Idle
        # "Initialization Macro\n(This is called once, when the VI starts)"
        n183 = call <vilib>:"Add State(s) to Queue__JKI_lib_State_Machine.vi"("State(s) in Front (\"\")"=w400, "State(s) in (\"\")"=w404) -> ("States Out"=w403:string)  [unwired: 13 in]
      }
      frame "Macro: Exit" {
        # "Exit Macro\n(This is called once, when the VI exits)"
        n184 = Unbundle By Name(w411) -> ("Core.Close Panel on Exit?"=w410:bool)
        n185 = Select(t="UI: Front Panel State >> Close", s=w410, f="") -> (s? t:f=w407:string)
        n186 = call <vilib>:"Add State(s) to Queue__JKI_lib_State_Machine.vi"("State(s) in (\"\")"=w407, "State(s) at Back (\"\")"="Data: Cleanup\nExit") -> ("States Out"=w405:string)  [unwired: 13 in]
        n187 = call <vilib>:"Add State(s) to Queue__JKI_lib_State_Machine.vi"("State(s) in Front (\"\")"=w405, "State(s) in (\"\")"=w414) -> ("States Out"=w413:string)  [unwired: 13 in]
      }
      frame "---------- VIPM ----------" {
        # "Template Separator\n(You can make a copy of, or modify, this frame)"
        n188 = call <vilib>:"Add State(s) to Queue__JKI_lib_State_Machine.vi"("State(s) in (\"\")"=w418) -> ("States Out"=w417:string)  [unwired: 14 in]
      }
      frame "VIPM: Open File" {
        # "Your code here.\n(You can make a copy of, or modify, this frame)"
        n189 = Unbundle By Name(w429) -> ("selected path"=w419:path)
        n190 = Format Into String(format string="cmd /c explorer.exe \"%s\"", error in=w423, w419) -> (resulting string=w427:string, error out=w425:errorcluster)  [unwired: 1 in]
        n191 = Strip Path(path=w419) -> (name=w421:string)  [unwired: 1 out]
        n192 = call <vilib>:"System Exec.vi"("run minimized? (F)"=TRUE, "error in (no error)"=w425, "command line"=w427) -> ("error out"=w424:errorcluster)  [unwired: 5 in, 3 out]
        n193 = Format Into String(format string="Opening \"%s\"...", w421) -> (resulting string=w422:string)  [unwired: 2 in, 1 out]
        n194 = local write "Status"(w422) -> ()
        n195 = call <vilib>:"Add State(s) to Queue__JKI_lib_State_Machine.vi"("State(s) in (\"\")"=w431) -> ("States Out"=w430:string)  [unwired: 14 in]
      }
      frame "VIPM: Preview VIPB" {
        # "Your code here.\n(You can make a copy of, or modify, this frame)"
        n196 = Unbundle By Name(w441) -> ("vipb paths"=w435:path[], "selected path"=w437:path)
        n197 = local read "ALL"() -> (w432:bool)
        n198 = Build Array(w437) -> (w434:path[])
        n199 = Select(t=w435, s=w432, f=w434) -> (s? t:f=w436:path[])
        n200 = for {
          tunnel: w436 -> [w447] mode=indexing
          tunnel: [w450] -> w440
          tunnel: w439 -> [w449]
          tunnel: [w448] -> w438 mode=indexing
          n201 = Strip Path(path=w447) -> (name=w444:string)  [unwired: 1 out]
          n202 = Format Into String(format string="Reading \"%s\"...", w444) -> (resulting string=w446:string)  [unwired: 2 in, 1 out]
          n203 = call <vilib>:"Read VI Package Build Spec_vipm_api.vi"("error in (no error)"=w449, "Path to VIPB File"=w447) -> ("error out"=w450:errorcluster, "VI Package Build Spec Data"=w448:T7)  [unwired: 8 in]
          n204 = local write "Status"(w446) -> ()
        }
        n205 = call "Format Build Spec Summary.vi"("Build Spec [] in"=w438) -> ("VIPB Preview"=w433:string)  [unwired: 10 in]
        n206 = local write "Status"(w433) -> ()
        n207 = call <vilib>:"Add State(s) to Queue__JKI_lib_State_Machine.vi"("State(s) in (\"\")"=w443) -> ("States Out"=w442:string)  [unwired: 14 in]
      }
      frame "VIPM: Increment Patch" {
        # "Your code here.\n(You can make a copy of, or modify, this frame)"
        n208 = Unbundle By Name(w460) -> ("vipb paths"=w456:path[], "selected path"=w458:path)
        n209 = local read "ALL"() -> (w451:bool)
        n210 = Build Array(w458) -> (w455:path[])
        n211 = Select(t=w456, s=w451, f=w455) -> (s? t:f=w457:path[])
        n212 = for {
          tunnel: w457 -> [w466] mode=indexing
          tunnel: w452 -> [w476]
          tunnel: [w467] -> w459 mode=indexing
          tunnel: [w465] -> w453
          n213 = call <vilib>:"Read VI Package Build Spec_vipm_api.vi"("error in (no error)"=w476, "Path to VIPB File"=w466) -> ("error out"=w472:errorcluster, "VI Package Build Spec Data"=w471:T7)  [unwired: 8 in]
          n214 = Unbundle By Name(w471) -> ("Package Version.patch"=w463:u32)
          n215 = Strip Path(path=w466) -> (name=w473:string)  [unwired: 1 out]
          n216 = Increment(x=w463) -> (x+1=w470:u32)
          n217 = Format Into String(format string="Updating \"%s\"...", w473) -> (resulting string=w475:string)  [unwired: 2 in, 1 out]
          n218 = Bundle By Name(cluster=w471, "Package Version.patch"=w470, "Package Version.build"=u32 1) -> (w469:T7)
          n219 = local write "Status"(w475) -> ()
          n220 = call <vilib>:"Write VI Package Build Spec_vipm_api.vi"("error in (no error)"=w472, "VI Package Build Spec Data"=w469, "Path to VIPB File"=w466) -> ("error out"=w468:errorcluster)  [unwired: 8 in]
          n221 = call <vilib>:"Read VI Package Build Spec_vipm_api.vi"("error in (no error)"=w468, "Path to VIPB File"=w466) -> ("error out"=w465:errorcluster, "VI Package Build Spec Data"=w467:T7)  [unwired: 8 in]
        }
        n222 = call "Format Build Spec Summary.vi"("Build Spec [] in"=w459) -> ("VIPB Preview"=w454:string)  [unwired: 10 in]
        n223 = local write "Status"(w454) -> ()
        n224 = call <vilib>:"Add State(s) to Queue__JKI_lib_State_Machine.vi"("State(s) in (\"\")"=w462) -> ("States Out"=w461:string)  [unwired: 14 in]
      }
      frame "VIPM: Clear Notes" {
        # "Your code here.\n(You can make a copy of, or modify, this frame)"
        n225 = Unbundle By Name(w486) -> ("vipb paths"=w482:path[], "selected path"=w484:path)
        n226 = local read "ALL"() -> (w477:bool)
        n227 = Build Array(w484) -> (w481:path[])
        n228 = Select(t=w482, s=w477, f=w481) -> (s? t:f=w483:path[])
        n229 = for {
          tunnel: w483 -> [w491] mode=indexing
          tunnel: w478 -> [w500]
          tunnel: [w492] -> w485 mode=indexing
          tunnel: [w490] -> w479
          n230 = call <vilib>:"Read VI Package Build Spec_vipm_api.vi"("error in (no error)"=w500, "Path to VIPB File"=w491) -> ("error out"=w496:errorcluster, "VI Package Build Spec Data"=w495:T7)  [unwired: 8 in]
          n231 = Bundle By Name(cluster=w495, "Release Notes - Change Log"="") -> (w494:T7)
          n232 = Strip Path(path=w491) -> (name=w497:string)  [unwired: 1 out]
          n233 = Format Into String(format string="Updating \"%s\"...", w497) -> (resulting string=w499:string)  [unwired: 2 in, 1 out]
          n234 = local write "Status"(w499) -> ()
          n235 = call <vilib>:"Write VI Package Build Spec_vipm_api.vi"("error in (no error)"=w496, "VI Package Build Spec Data"=w494, "Path to VIPB File"=w491) -> ("error out"=w493:errorcluster)  [unwired: 8 in]
          n236 = call <vilib>:"Read VI Package Build Spec_vipm_api.vi"("error in (no error)"=w493, "Path to VIPB File"=w491) -> ("error out"=w490:errorcluster, "VI Package Build Spec Data"=w492:T7)  [unwired: 8 in]
        }
        n237 = call "Format Build Spec Summary.vi"("Build Spec [] in"=w485) -> ("VIPB Preview"=w480:string)  [unwired: 10 in]
        n238 = local write "Status"(w480) -> ()
        n239 = call <vilib>:"Add State(s) to Queue__JKI_lib_State_Machine.vi"("State(s) in (\"\")"=w488) -> ("States Out"=w487:string)  [unwired: 14 in]
      }
      frame "VIPM: Append Notes" {
        # "Your code here.\n(You can make a copy of, or modify, this frame)"
        n240 = Unbundle By Name(w510) -> ("vipb paths"=w506:path[], "selected path"=w508:path)
        n241 = local read "ALL"() -> (w501:bool)
        n242 = Build Array(w508) -> (w505:path[])
        n243 = Select(t=w506, s=w501, f=w505) -> (s? t:f=w507:path[])
        n244 = for {
          tunnel: w507 -> [w521] mode=indexing
          tunnel: w502 -> [w529]
          tunnel: [w522] -> w509 mode=indexing
          tunnel: [w520] -> w503
          n245 = call <vilib>:"Read VI Package Build Spec_vipm_api.vi"("error in (no error)"=w529, "Path to VIPB File"=w521) -> ("error out"=w525:errorcluster, "VI Package Build Spec Data"=w519:T7)  [unwired: 8 in]
          n246 = Unbundle By Name(w519) -> ("Release Notes - Change Log"=w514:string)
          n247 = Strip Path(path=w521) -> (name=w526:string)  [unwired: 1 out]
          n248 = Concatenate Strings(w514, "\n", "Release Notes") -> (w513:string)
          n249 = Format Into String(format string="Updating \"%s\"...", w526) -> (resulting string=w528:string)  [unwired: 2 in, 1 out]
          n250 = Empty String/Path?(string/path=w514) -> (empty?=w518:bool)
          n251 = Select(t="Release Notes", s=w518, f=w513) -> (s? t:f=w517:string)
          n252 = Bundle By Name(cluster=w519, "Release Notes - Change Log"=w517) -> (w524:T7)
          n253 = local write "Status"(w528) -> ()
          n254 = call <vilib>:"Write VI Package Build Spec_vipm_api.vi"("error in (no error)"=w525, "VI Package Build Spec Data"=w524, "Path to VIPB File"=w521) -> ("error out"=w523:errorcluster)  [unwired: 8 in]
          n255 = call <vilib>:"Read VI Package Build Spec_vipm_api.vi"("error in (no error)"=w523, "Path to VIPB File"=w521) -> ("error out"=w520:errorcluster, "VI Package Build Spec Data"=w522:T7)  [unwired: 8 in]
        }
        n256 = call "Format Build Spec Summary.vi"("Build Spec [] in"=w509) -> ("VIPB Preview"=w504:string)  [unwired: 10 in]
        n257 = local write "Status"(w504) -> ()
        n258 = call <vilib>:"Add State(s) to Queue__JKI_lib_State_Machine.vi"("State(s) in (\"\")"=w512) -> ("States Out"=w511:string)  [unwired: 14 in]
      }
      frame "VIPM: Build VIPB" {
        # "Template Separator\n(You can make a copy of, or modify, this frame)"
        n259 = Unbundle By Name(w535) -> ("vipb paths"=w540:path[], "selected path"=w542:path)
        n260 = local read "ALL"() -> (w530:bool)
        n261 = Build Array(w542) -> (w539:path[])
        n262 = Select(t=w540, s=w530, f=w539) -> (s? t:f=w541:path[])
        n263 = for {
          tunnel: w541 -> [w545] mode=indexing
          tunnel: [w551] -> w538
          tunnel: w537 -> [w550]
          tunnel: [w549] -> w534 mode=indexing
          n264 = Strip Path(path=w545) -> (name=w546:string)  [unwired: 1 out]
          n265 = Format Into String(format string="Building \"%s\"...", w546) -> (resulting string=w548:string)  [unwired: 2 in, 1 out]
          n266 = local write "Status"(w548) -> ()
          n267 = call <vilib>:"Build VI Package_vipm_api.vi"("error in (no error)"=w550, "Path to VIPB File"=w545) -> ("error out"=w551:errorcluster, "Build Output"=w549:path)  [unwired: 8 in]
        }
        n268 = call <vilib>:"Build State String with Arguments__JKI_lib_State_Machine.vi"("Arguments (\"\")"=w532, "State"="VIPM: Preview VIPB" ("State(s) in Front (\"\")")) -> ("State with Arguments"=w533:string)  [unwired: 4 in]
        n269 = Bundle By Name(cluster=w535, "vip paths"=w534) -> (w536:T4)
        n270 = call <vilib>:"Add State(s) to Queue__JKI_lib_State_Machine.vi"("State(s) in Front (\"\")"=w533, "State(s) in (\"\")"=w544) -> ("States Out"=w543:string)  [unwired: 13 in]
      }
      frame "VIPM: Publish VIPB" {
        # "Template Separator\n(You can make a copy of, or modify, this frame)"
        n271 = Unbundle By Name(w555) -> ("vip paths"=w554:path[])
        n272 = call <vilib>:"List VIPM Managed Repositories_vipm_api.vi"("error in (no error)"=w552) -> ("Managed Repositories Info"=w556:T9[], "error out"=w557:errorcluster)  [unwired: 13 in]
        n273 = Index Array(array=w556) -> (element=w558:T9)  [unwired: 1 in]
        n274 = Unbundle By Name(w558) -> ("Repository Name"=w559:string)
        n275 = call <vilib>:"Publish VI Packages to Repository_vipm_api.vi"("error in (no error)"=w557, "Repository Name"=w559, "Packages to publish to Repository Library (vip,ogp)"=w554) -> ("error out"=w553:errorcluster)  [unwired: 7 in, 1 out]
        n276 = call <vilib>:"Add State(s) to Queue__JKI_lib_State_Machine.vi"("State(s) in (\"\")"=w561) -> ("States Out"=w560:string)  [unwired: 14 in]
      }
    }
  }
